vi "Explain LabView Error Code.vi"(1 "Error Code":i32) -> (0 "Error Text":string)   [LabVIEW 2019, in "Error.lvclass"]
uses:
  Error.lvclass
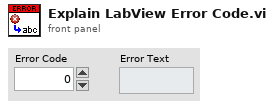
[diagram p1: front panel]
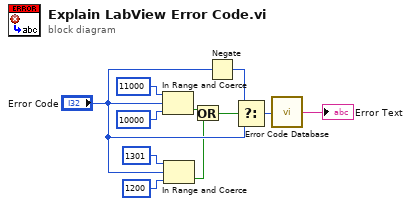
[diagram p0: block diagram]
diagram:
  n1 = In Range and Coerce(upper limit=11000, x="Error Code", lower limit=10000) -> (In Range?=w3:bool)  [unwired: 1 out]
  n2 = In Range and Coerce(upper limit=1301, x="Error Code", lower limit=1200) -> (In Range?=w2:bool)  [unwired: 1 out]
  n3 = Or(x=w3, y=w2) -> (x .or. y?=w4:bool)
  n4 = Negate(x="Error Code") -> (-x=w1:i32)
  n5 = Select(t=w1, s=w4, f="Error Code") -> (s? t:f=w5:i32)
  n6 = call <vilib>:"Error Code Database.vi"("Error Code"=w5) -> ("Error Text"=→"Error Text":string)
